vi "potCalculations.vi"(11 "Voltage in":dbl) -> (3 "distance out":dbl)   [LabVIEW 2015]
uses:
  Robot Global Data.vi
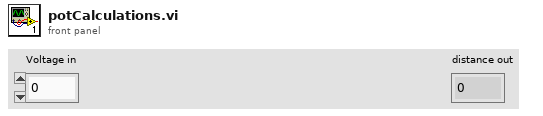
[diagram p1: front panel]
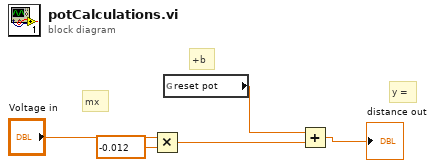
[diagram p0: block diagram]
diagram:
  # "+b"
  # "mx"
  # "y ="
  n1 = Multiply(x="Voltage in", y=-0.012) -> (x*y=w4:dbl)
  n2 = global read "Robot Global Data.vi" "reset pot"() -> (w1:dbl)
  n3 = Add(x=w1, y=w4) -> (x+y=→"distance out":dbl)
